vi "Integrate_diag.vi"(0 "Processed LD values":dbl[](array[numeric]), 1 "Processed LD time values":dbl[](array[numeric]), 5 "Cutoff Frequency":dbl, 9 "Window (s)":dbl, 12 "Ref Sine":dbl[](array[numeric]), 13 "Ref Cosine":dbl[](array[numeric])) -> (3 "Lockin Theta":cluster{dbl[], "Result":dbl[]}, 4 "Numeric":dbl, 6 "Lock in X,Y,R (Vrms) time":cluster{dbl[], "Result":dbl[]}[](array[cluster]), 8 "LockIn Theta Array":dbl[](array[numeric]), 10 "LockIn R (Vrms) array":dbl[](array[numeric]), 14 "LockIN R (cont/disc)":waveform(dbl)[](graph), 15 "LockIn R (Vrms)":cluster{dbl[], "Result":dbl[]})   [LabVIEW 2013]
uses:
  <vilib>/Analysis/8numeric.llb/1D Numeric Integration.vi
  <vilib>/express/express arith-compare/Formula/XNode/ExpressFormulaBlockNode.xnode
  <vilib>/Analysis/NI_AALPro.lvlib
  <vilib>/Analysis/NI_AALBase.lvlib
panel:
  out "X":dbl[](graph)
  out "Y":dbl[](graph)
  out "Waveform Graph 2":dbl[](graph)
  out "Phase (deg)":waveform(dbl)(graph)
  out "standard deviation 2":dbl format="%0.2f"
  out "mean 2":dbl format="%0.2f"
  out "standard deviation":dbl format="%0.5f"
  out "mean":dbl format="%0.5f"
  out "theta":dbl[](array[numeric])
  out "r":dbl[](array[numeric])
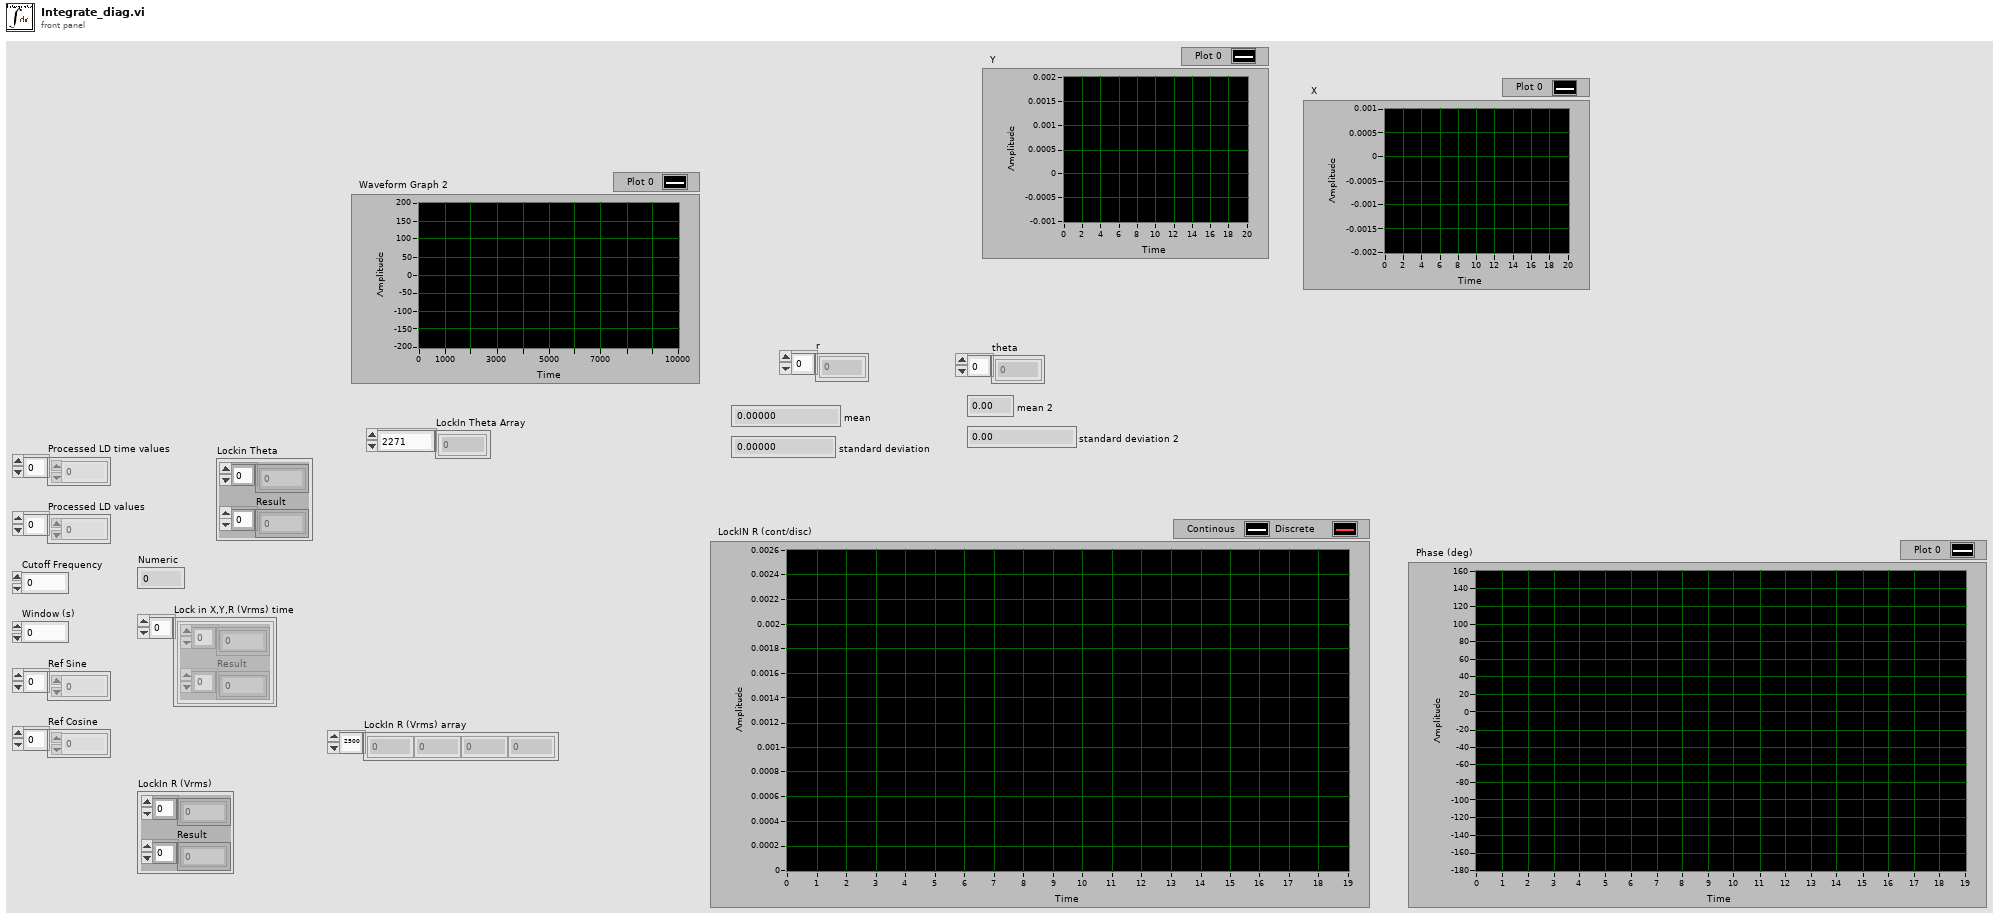
[diagram p1: front panel]
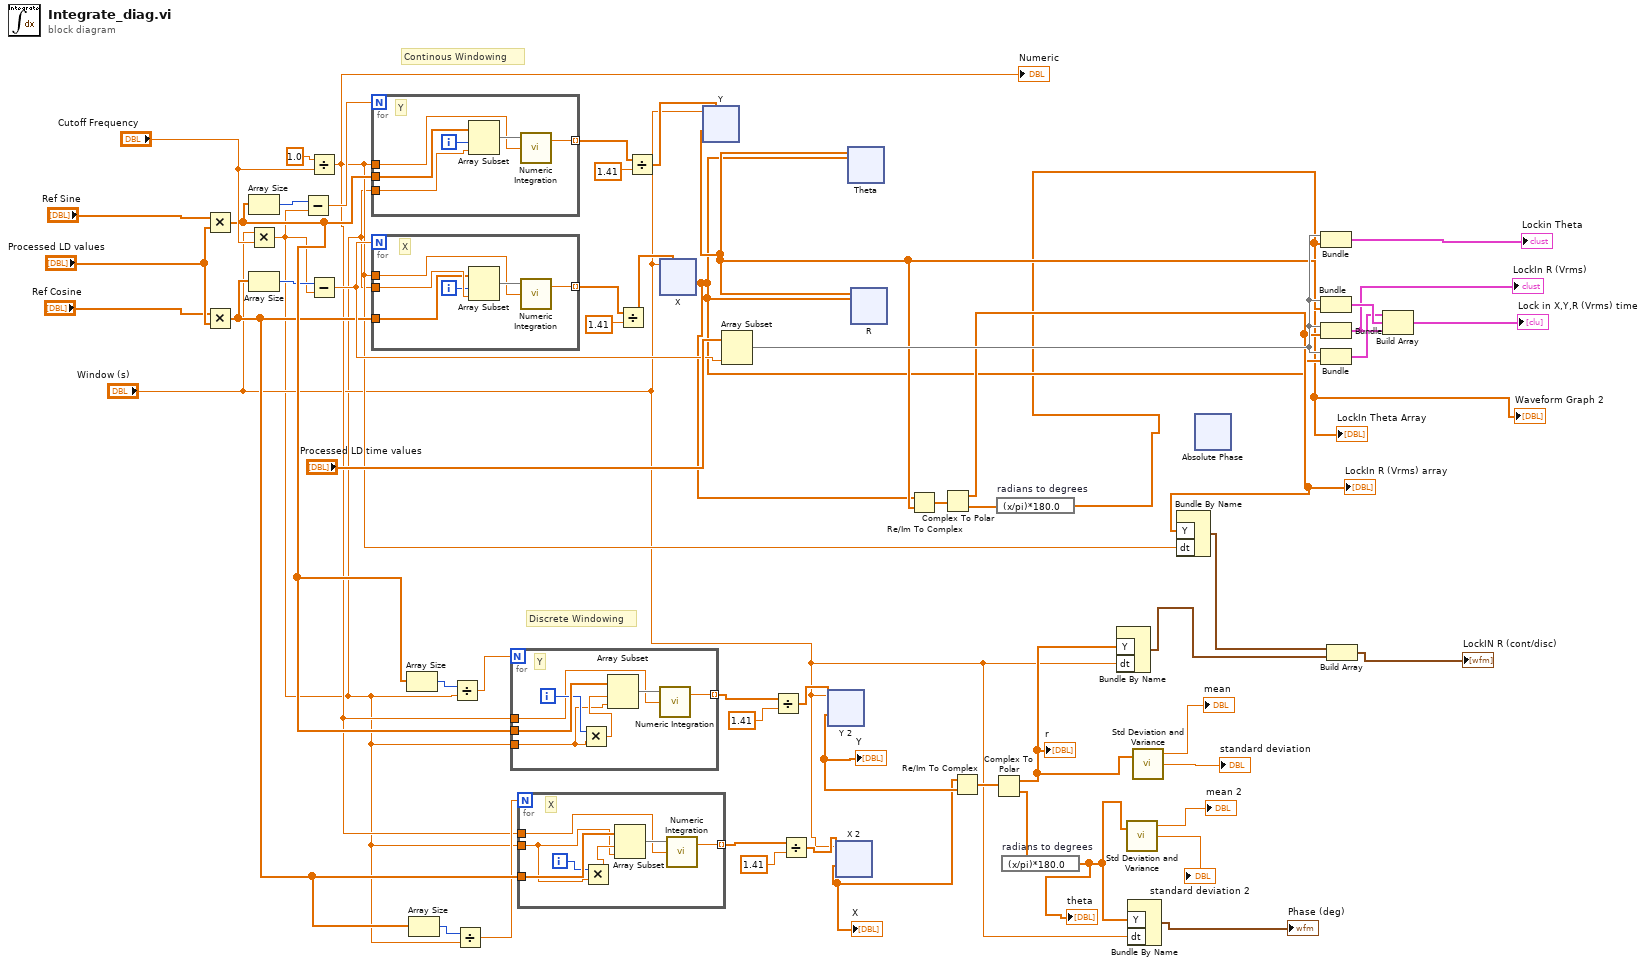
[diagram p0: block diagram]
diagram:
  # "Continous Windowing"
  # "Discrete Windowing"
  n1 = Multiply(x="Ref Sine", y="Processed LD values") -> (x*y=w35:dbl[])
  n2 = Multiply(x="Ref Cosine", y="Processed LD values") -> (x*y=w34:dbl[])
  n3 = Array Size(array=w35) -> (size(s)=w9:i32)
  n4 = Multiply(x="Window (s)", y="Cutoff Frequency") -> (x*y=w7:dbl)
  n5 = Array Size(array=w34) -> (size(s)=w8:i32)
  n6 = Subtract(x=w9, y=w7) -> (x-y=w45:dbl)
  n7 = Divide(x=1.0, y="Cutoff Frequency") -> (x/y=w11:dbl)
  "Numeric" <- w11
  n8 = Subtract(x=w8, y=w7) -> (x-y=w44:dbl)
  n9 = for {
    N: w45 -> [_]
    tunnel: w35 -> [w63]
    tunnel: w7 -> [w62]
    tunnel: [w59] -> w39 mode=indexing
    tunnel: w11 -> [w58]
    i -> [w61]
    # "Y"
    n10 = Array Subset(array=w63, index=w61, length=w62) -> (w60:dbl[])
    n11 = call-poly <vilib>:"Numeric Integration.vi"("dt"=w58, "Input Array"=w60) -> ("result"=w59:dbl)  [unwired: 1 in, 1 out]
  }
  n12 = for {
    N: w44 -> [_]
    tunnel: w34 -> [w67]
    tunnel: w7 -> [w69]
    tunnel: [w65] -> w42 mode=indexing
    tunnel: w11 -> [w64]
    i -> [w68]
    # "X"
    n13 = Array Subset(array=w67, index=w68, length=w69) -> (w66:dbl[])
    n14 = call-poly <vilib>:"Numeric Integration.vi"("dt"=w64, "Input Array"=w66) -> ("result"=w65:dbl)  [unwired: 1 in, 1 out]
  }
  n15 = Array Size(array=w35) -> (size(s)=w33:i32)
  n16 = Array Size(array=w34) -> (size(s)=w32:i32)
  n17 = Divide(x=w33, y=w7) -> (x/y=w31:dbl)
  n18 = Divide(x=w32, y=w7) -> (x/y=w30:dbl)
  n19 = for {
    N: w31 -> [_]
    tunnel: w35 -> [w76]
    tunnel: w7 -> [w70]
    tunnel: [w74] -> w29 mode=indexing
    tunnel: w11 -> [w71]
    i -> [w72]
    # "Y"
    n20 = Multiply(x=w72, y=w70) -> (x*y=w73:dbl)
    n21 = Array Subset(array=w76, index=w73, length=w70) -> (w75:dbl[])
    n22 = call-poly <vilib>:"Numeric Integration.vi"("dt"=w71, "Input Array"=w75) -> ("result"=w74:dbl)  [unwired: 1 in, 1 out]
  }
  n23 = for {
    N: w30 -> [_]
    tunnel: w34 -> [w83]
    tunnel: w7 -> [w77]
    tunnel: [w81] -> w26 mode=indexing
    tunnel: w11 -> [w80]
    i -> [w79]
    # "X"
    n24 = Multiply(x=w79, y=w77) -> (x*y=w78:dbl)
    n25 = Array Subset(array=w83, index=w78, length=w77) -> (w82:dbl[])
    n26 = call-poly <vilib>:"Numeric Integration.vi"("dt"=w80, "Input Array"=w82) -> ("result"=w81:dbl)  [unwired: 1 in, 1 out]
  }
  n27 = Divide(x=w42, y=1.41) -> (x/y=w41:dbl[])
  n28 = Divide(x=w39, y=1.41) -> (x/y=w38:dbl[])
  n29 = xnode "X"("X1"="Window (s)", "X2"=w41) -> ("Result"=w12:dbl[])  [unwired: 1 in, 1 out]
  n30 = xnode "Y"("X1"="Window (s)", "X2"=w38) -> ("Result"=w36:dbl[])  [unwired: 1 in, 1 out]
  n31 = Array Subset(array="Processed LD time values", length=w44) -> (w48:dbl[])  [unwired: 1 in]
  n32 = Divide(x=w29, y=1.41) -> (x/y=w20:dbl[])
  n33 = Divide(x=w26, y=1.41) -> (x/y=w19:dbl[])
  n34 = xnode "Y 2"("X1"="Window (s)", "X2"=w20) -> ("Result"=w2:dbl[])  [unwired: 1 in, 1 out]
  "Y" <- w2
  n35 = xnode "X 2"("X1"="Window (s)", "X2"=w19) -> ("Result"=w1:dbl[])  [unwired: 1 in, 1 out]
  "X" <- w1
  n36 = xnode "Theta"("X1"=w36, "X2"=w12) -> ()  [unwired: 1 in, 2 out]
  n37 = xnode "R"("X1"=w36, "X2"=w12) -> ()  [unwired: 1 in, 2 out]
  n38 = Re/Im To Complex(1:w36, 2:w12) -> (0:w37:cdb[])
  n39 = Complex To Polar(r * e^(i*theta)=w37) -> (r=w16:dbl[], theta=w6:dbl[])
  "LockIn R (Vrms) array" <- w16
  n40 = Re/Im To Complex(1:w2, 2:w1) -> (0:w25:cdb[])
  n41 = Complex To Polar(r * e^(i*theta)=w25) -> (r=w18:dbl[], theta=w5:dbl[])
  "r" <- w18
  n42 = expression code="(x/pi)*180.0" "radians to degrees"(w6) -> (w3:dbl[])
  "LockIn Theta Array" <- w3
  "Waveform Graph 2" <- w3
  n43 = expression code="(x/pi)*180.0" "radians to degrees"(w5) -> (w4:dbl[])
  "theta" <- w4
  n44 = Bundle By Name("Y"=w18, "dt"="Window (s)") -> (w14:waveform(dbl))  [unwired: 1 in]
  n45 = call <vilib>:"Std Deviation and Variance.vi"("X"=w4) -> ("mean"=→"mean 2":dbl, "standard deviation"=→"standard deviation 2":dbl)  [unwired: 1 in, 1 out]
  n46 = Bundle By Name("Y"=w4, "dt"="Window (s)") -> (→"Phase (deg)":waveform(dbl))  [unwired: 1 in]
  n47 = call <vilib>:"Std Deviation and Variance.vi"("X"=w18) -> ("mean"=→"mean":dbl, "standard deviation"=→"standard deviation":dbl)  [unwired: 1 in, 1 out]
  n48 = Bundle By Name("Y"=w16, "dt"=w11) -> (w15:waveform(dbl))  [unwired: 1 in]
  n49 = xnode "Absolute Phase"() -> ()  [unwired: 2 in, 2 out]
  n50 = Bundle(w48, w3) -> (→"Lockin Theta":cluster{dbl[], dbl[]})  [unwired: 1 in]
  n51 = Bundle(w48, "Result"=w36) -> (w53:cluster{dbl[], "Result":dbl[]})  [unwired: 1 in]
  n52 = Bundle(w48, w16) -> (w49:cluster{dbl[], dbl[]})  [unwired: 1 in]
  "LockIn R (Vrms)" <- w49
  n53 = Bundle(w48, "Result"=w12) -> (w52:cluster{dbl[], "Result":dbl[]})  [unwired: 1 in]
  n54 = Build Array(w15, w14) -> (→"LockIN R (cont/disc)":waveform(dbl)[])
  n55 = Build Array(w52, w53, w49) -> (→"Lock in X,Y,R (Vrms) time":cluster{dbl[], "Result":dbl[]}[])
